vi "Initialize.vi"(7 "Process ID":string, 8 "error in (no error)":errorcluster, 11 "Process in":refnum<class "Process.lvclass">) -> (0 "error out":errorcluster, 3 "Process out":refnum<class "Process.lvclass">)   [LabVIEW 2019, in "TelemetryAsync Engine.lvlib" / "Process.lvclass"]
uses:
  Process.lvclass
  TypeDefs/Message.ctl
  TypeDefs/Update.ctl
  Process.lvclass/Process.ctl
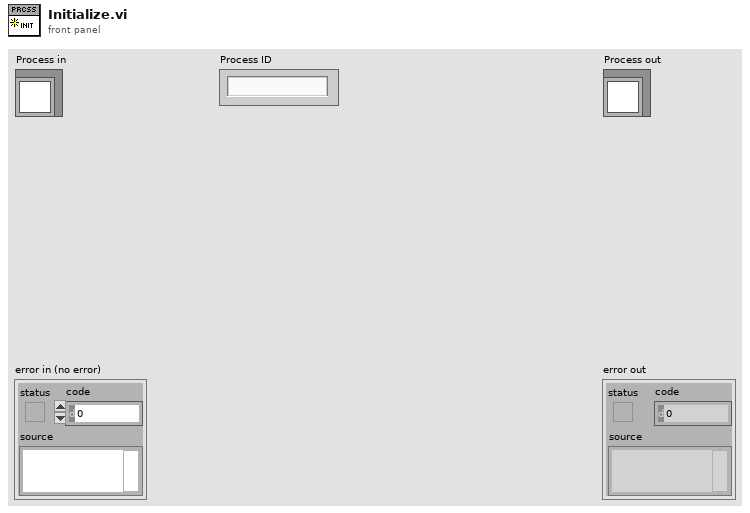
[diagram p1: front panel]
types:
  T1 = typedef "TelemetryAsync Engine.lvlib/Process.lvclass/Update.ctl" = cluster{"Update Message":string, "Payload":variant}
  T2 = typedef "TelemetryAsync Engine.lvlib/Process.lvclass/Message.ctl" = cluster{"Command":string, "Payload":variant}
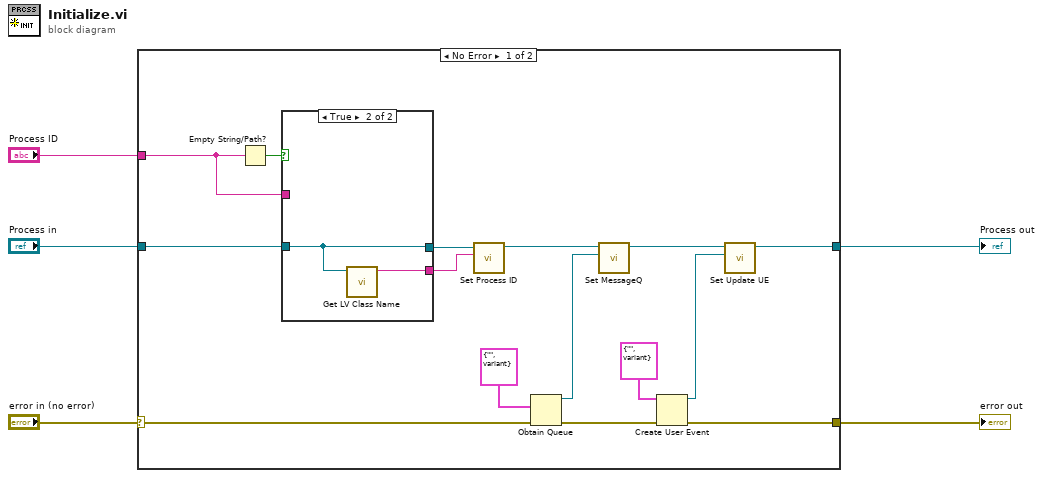
[diagram p0: block diagram]
diagram:
  n1 = case shown="No Error" "error in (no error)" {
    selector: "error in (no error)" -> [w20 w26]
    tunnel: [w12 w26] -> w4
    tunnel: [w7 w25] -> w2
    tunnel: "Process in" -> [w6 w25]
    tunnel: "Process ID" -> [w10 _]
    frame No Error {
      n2 = Empty String/Path?(string/path=w10) -> (empty?=w11:bool)
      n3 = case shown="True" w11 {
        tunnel: w10 -> [w22 _]
        tunnel: w6 -> [w21 w24]
        tunnel: [w21 w24] -> w9
        tunnel: [w22 w23] -> w8
        frame False {
        }
        frame True {
          n4 = call <vilib>:"Get LV Class Name.vi"("object"=w24) -> ("class name"=w23:string)  [unwired: 9 in, 1 out]
        }
      }
      n5 = call "Set Process ID.vi"("Process ID"=w8, "CD_Process in"=w9) -> ("CD_Process out"=w17:refnum<class "Process.lvclass">)  [unwired: 9 in]
      n6 = Obtain Queue(element data type=T2 {"Command"="", "Payload"=variant}, error in (no error)=w20) -> (queue out=w18:refnum<queue>, error out=w16:errorcluster)  [unwired: 3 in, 1 out]
      n7 = call "Set MessageQ.vi"("MessageQ"=w18, "CD_Process in"=w17) -> ("CD_Process out"=w14:refnum<class "Process.lvclass">)  [unwired: 9 in]
      n8 = Create User Event(user event datatype=T1 {"Update Message"="", "Payload"=variant} ("Update"), error in=w16) -> (user event=w13:refnum<user-event>, error out=w12:errorcluster)
      n9 = call "Set Update UE.vi"("Update UE"=w13, "CD_Process in"=w14) -> ("CD_Process out"=w7:refnum<class "Process.lvclass">)  [unwired: 9 in]
    }
    frame Error {
    }
  }
  "error out" <- w4
  "Process out" <- w2
